vi "Servo MSMT LTE Configure Fetch Step.vi"(8 "error in (no error)":errorcluster, 10 "LTE Standard In":string, 11 "Servo MSMT in":refnum<class "Servo MSMT.lvclass">) -> (0 "error out":errorcluster, 3 "Servo MSMT out":refnum<class "Servo MSMT.lvclass">)   [LabVIEW 2018, in "Servo MSMT.lvlib" / "Servo MSMT.lvclass"]
uses:
  Servo MSMT.lvclass
  C:/Sequence Automation/Plugins/Measurement Interface.lvlibp/Measurement Interface.lvclass
  Plugins/Measurement Interface.lvlibp/Private Methods/Measurement Name/Read Measurement Name.vi
  Plugins/Measurement Interface.lvlibp/Private Methods/Engine Reference/Read Engine Reference.vi
  Plugins/Measurement Interface.lvlibp/Public Methods/Sequence Reference/Read Sequence Reference.vi
  Plugins/TestStand API Tools (TSAT).lvlibp/Step Actions/TSAT Step Actions.lvlib
  Plugins/TestStand API Tools (TSAT).lvlibp/Sequence Actions/TSAT Sequence Actions.lvlib
  Plugins/Measurement Interface.lvlibp/Measurement Interface.lvclass
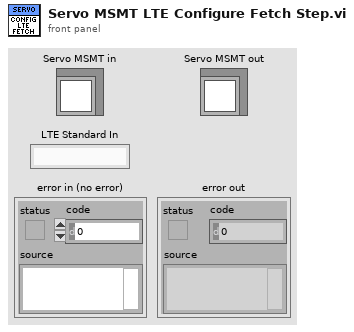
[diagram p1: front panel]
types:
  T1 = typedef "TestStand API Tools (TSAT).lvlibp/TSAT Evaluation Actions.lvlib/TSAT Evaluation.ctl" = cluster{"Test Name":string, "Pin":string, "Units":string, "SI Scaling":T2, "Test Number":i32, "Published Data Id":string, "Low Limit":dbl, "High Limit":dbl, "Export Data Location":string, "Software Bin":i64, "Evaluation Type":T3, "Test Data Source":string}
  T2 = typedef "TestStand API Tools (TSAT).lvlibp/TSAT Evaluation Actions.lvlib/TSAT Eval SI Unit Scaling.ctl" = i16
  T3 = typedef "TestStand API Tools (TSAT).lvlibp/TSAT Evaluation Actions.lvlib/TSAT Evaluation Type.ctl" = enum16{"Numeric Limit", "Pass/Fail", "None"}
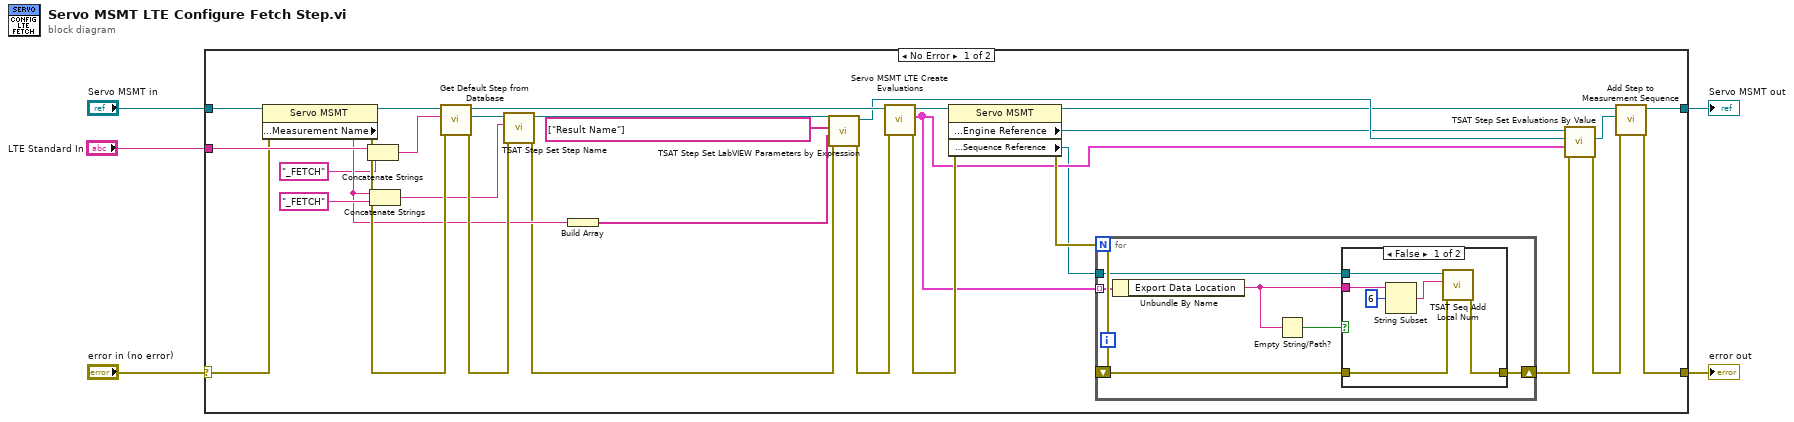
[diagram p0: block diagram]
diagram:
  n1 = case shown="No Error" "error in (no error)" {
    selector: "error in (no error)" -> [w29 w51]
    tunnel: [w19 w51] -> w4
    tunnel: [w18 w50] -> w2
    tunnel: "Servo MSMT in" -> [w36 w50]
    tunnel: "LTE Standard In" -> [w35 _]
    frame No Error {
      n2 = property class="Servo MSMT"(reference=w36, error in=w29) -> (reference out=w30:refnum<class "Servo MSMT.lvclass">, error out=w28:errorcluster, "Public Methods:Measurement Name"=w25:string)
      n3 = Concatenate Strings(w35, "_FETCH" ("string")) -> (w32:string)
      n4 = Concatenate Strings(w25, "_FETCH" ("string")) -> (w26:string)
      n5 = call "Get Default Step from Database.vi"("error in (no error)"=w28, "Default Step"=w32, "Measurement Interface in"=w30) -> ("error out"=w33:errorcluster, "Cloned Step"=w34:refnum<k7>, "Measurement Interface out"=w20:refnum<class "Servo MSMT.lvclass">)  [unwired: 6 in]
      n6 = call "TSAT Step Set Step Name.vi"("Error In"=w33, "Name"=w26, "Step In"=w34) -> ("Error Out"=w23:errorcluster, "Step Out"=w31:refnum<k7>)  [unwired: 7 in]
      n7 = Build Array(w25) -> (w24:string[])
      n8 = call "TSAT Step Set LabVIEW Parameters by Expression.vi"("Error In"=w23, "Value Expressions"=w24, "Parameters to Set"=string[] ["Result Name"], "Step In"=w31) -> ("Error Out"=w22:errorcluster, "Step Out"=w16:refnum<k7>)  [unwired: 6 in]
      n9 = call "Servo MSMT LTE Create Evaluations.vi"("error in (no error)"=w22, "Servo MSMT in"=w20) -> ("error out"=w10:errorcluster, "LTE Evaluations"=w7:T1[], "Servo MSMT out"=w14:refnum<class "Servo MSMT.lvclass">)  [unwired: 7 in]
      n10 = property class="Servo MSMT"(reference=w14, error in=w10) -> (reference out=w13:refnum<class "Servo MSMT.lvclass">, error out=w9:errorcluster, "Protected Methods:Engine Reference"=w12:refnum<k7>, "Public Methods:Sequence Reference"=w6:refnum<k7>)
      n11 = for {
        tunnel: w7 -> [w42] mode=indexing
        shift-right: [w40] -> w8
        shift-left: w9 -> [w41]
        tunnel: w6 -> [w39]
        n12 = Unbundle By Name(w42) -> ("Export Data Location"=w37:string)
        n13 = Empty String/Path?(string/path=w37) -> (empty?=w38:bool)
        n14 = case shown="False" w38 {
          tunnel: w41 -> [w46 w49]
          tunnel: [w45 w49] -> w40
          tunnel: w39 -> [w44 _]
          tunnel: w37 -> [w43 _]
          frame False {
            n15 = String Subset(string=w43, offset (0)=6) -> (substring=w47:string)  [unwired: 1 in]
            n16 = call "TSAT Seq Add Local Num.vi"("Error In"=w46, "Local Variable Name"=w47, "Sequence In"=w44) -> ("Error Out"=w45:errorcluster)  [unwired: 7 in, 1 out]
          }
          frame True {
          }
        }
      }
      n17 = call "TSAT Step Set Evaluations By Value.vi"("Error In"=w8, "Evaluation Data"=w7, "Step In"=w16, "Engine In"=w12) -> ("Error Out"=w15:errorcluster, "Step Out"=w17:refnum<k7>)  [unwired: 5 in, 1 out]
      n18 = call "Add Step to Measurement Sequence.vi"("error in (no error)"=w15, "Step to Add"=w17, "Measurement Interface in"=w13) -> ("error out"=w19:errorcluster, "Measurement Interface out"=w18:refnum<class "Servo MSMT.lvclass">)  [unwired: 7 in]
    }
    frame Error {
    }
  }
  "error out" <- w4
  "Servo MSMT out" <- w2
